vi "Write Destoying TS.vi"(8 "error in (no error)":errorcluster, 10 "Destroying":u64, 11 "CIFCorePlugin in":refnum<class "CIFCorePlugin.lvclass">) -> (0 "error out":errorcluster, 3 "CIFCorePlugin out":refnum<class "CIFCorePlugin.lvclass">)   [LabVIEW 2021, in "CIFCorePlugin.lvclass"]
doc: "Update the timestamp. Time is U64, absolute time in nS in the appropriate clockID configured for the plugin. If a 0 is wired it will automatically get the current time."
uses:
  CIFCorePlugin.lvclass
  CIFCorePlugin.lvclass/CIFCorePlugin.ctl
  CIFUtilities/CIFLogs/Typedef/Plugin State Commands.ctl
  CIFUtilities/CIFClocks/Time Conversion/LabVIEW Time to UTC Time.vi
  CIFUtilities/CIFClocks/SubVIs/Add Error.vi
  Common/Utilities/Append Error Location.vi
  CIFUtilities/CIFClocks/CIFClocks.lvlib
  CIFUtilities/CIFLogs/CIFLogs.lvlib
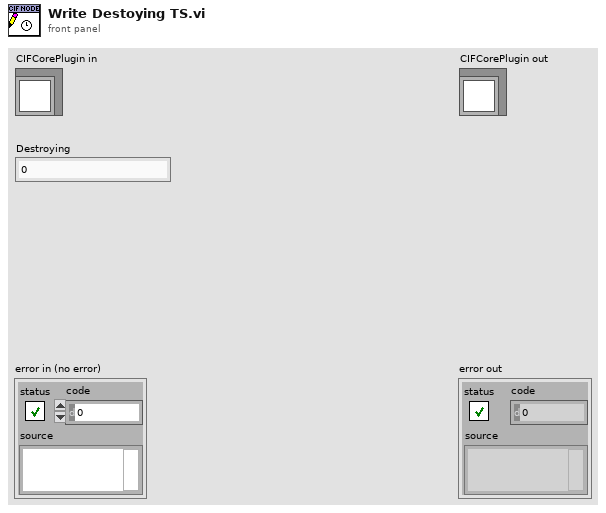
[diagram p1: front panel]
types:
  T1 = typedef "CIFLogs.lvlib/Plugin State Commands.ctl" = enum16{"Create", "Configure", "Run", "Pause", "Destroy"}
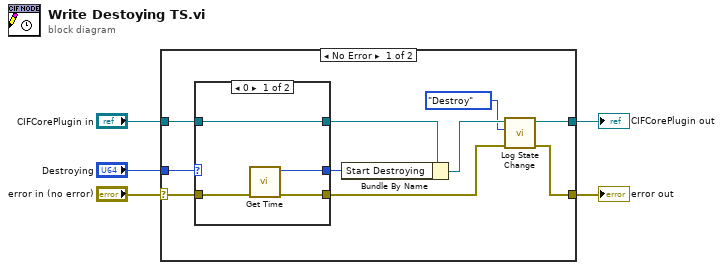
[diagram p0: block diagram]
diagram:
  n1 = case shown="No Error" "error in (no error)" {
    selector: "error in (no error)" -> [w14 w23]
    tunnel: [w6 w23] -> w4
    tunnel: [w8 w24] -> w2
    tunnel: "CIFCorePlugin in" -> [w13 w24]
    tunnel: "Destroying" -> [w15 _]
    frame No Error {
      n2 = case shown="0" w15 {
        selector: w15 -> [_ w21]
        tunnel: w14 -> [w18 w20]
        tunnel: w13 -> [w19 w22]
        tunnel: [w19 w22] -> w12
        tunnel: [w17 w21] -> w11
        tunnel: [w16 w20] -> w9
        frame 0 {
          n3 = call "Get Time.vi"("error in (no error)"=w18) -> ("error out"=w16:errorcluster, "Time (ns)"=w17:u64)  [unwired: 8 in, 1 out]
        }
        frame 1, Default {
        }
      }
      n4 = Bundle By Name(cluster=w12, "Start Destroying"=w11) -> (w10:refnum<class "CIFCorePlugin.lvclass">)
      n5 = call "Log State Change.vi"("error in (no error)"=w9, "Command"=Plugin_State_Commands."Destroy", "CIFCorePlugin in"=w10) -> ("error out"=w6:errorcluster, "CIFCorePlugin out"=w8:refnum<class "CIFCorePlugin.lvclass">)  [unwired: 7 in]
    }
    frame Error {
    }
  }
  "error out" <- w4
  "CIFCorePlugin out" <- w2
